vi "Seacrh and Replace String.vi"() -> ()   [LabVIEW 2020]
panel:
  out "Output String":string
  in  "Input String":string="My Self [Fisrt Name] [Last Name]  , My Age is [Age] , My Native Place is [Place]"
  in  "Stop Button":bool
  # "OverView :"
  # "Note :"
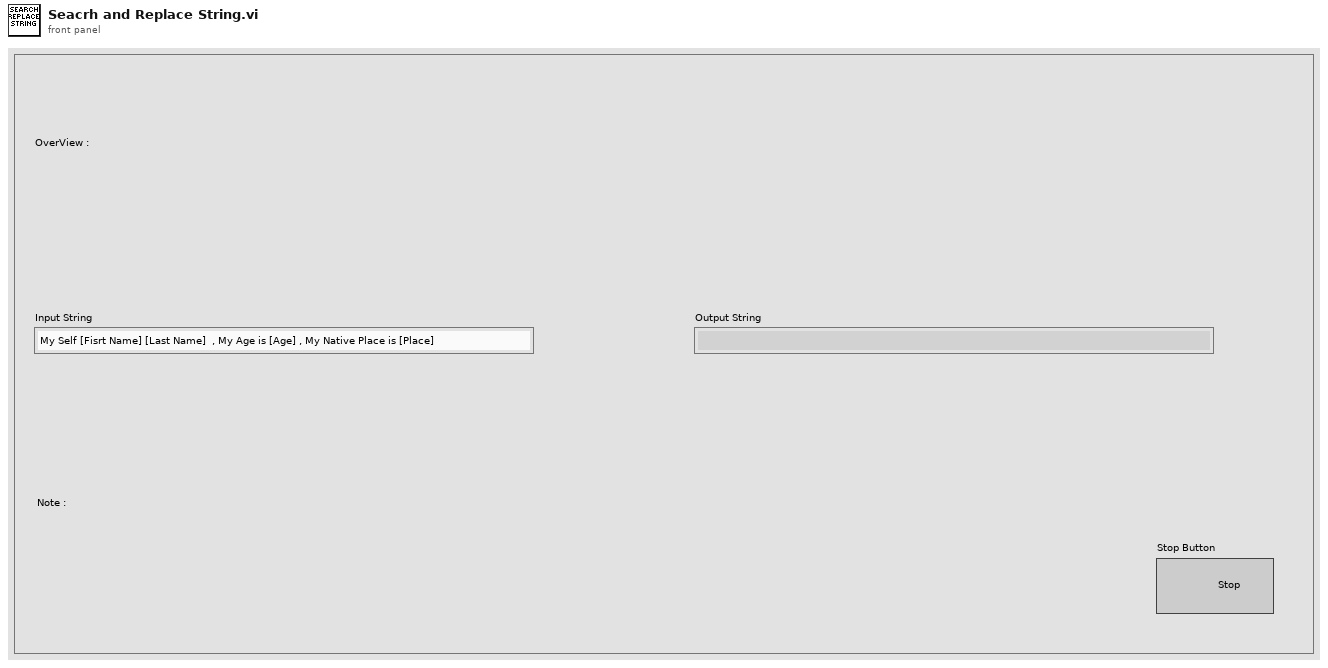
[diagram p1: front panel]
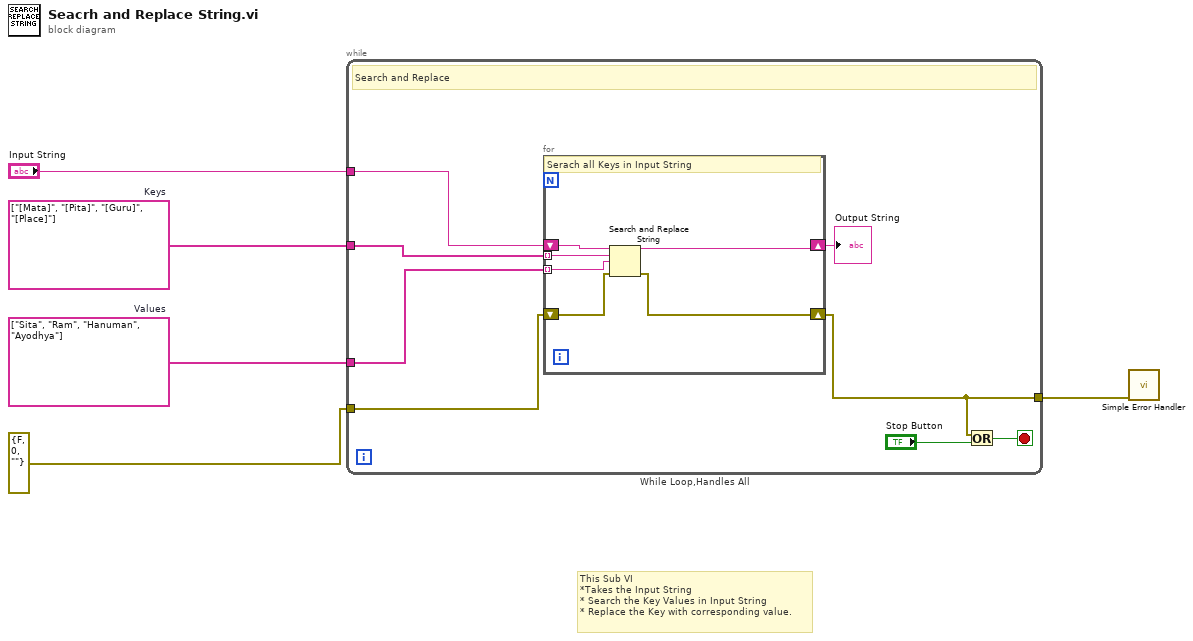
[diagram p0: block diagram]
diagram:
  w3 = string[] ["Sita", "Ram", "Hanuman", "Ayodhya"]  # Values
  w5 = string[] ["[Mata]", "[Pita]", "[Guru]", "[Place]"]  # Keys
  # "This Sub VI\n*Takes the Input String \n* Search the Key Values in Input String \n* Replace the Key with corresponding value."
  n1 = while "While Loop,Handles All" {
    tunnel: w5 -> [w10]
    tunnel: "Input String" -> [w11]
    tunnel: w3 -> [w9]
    tunnel: errorcluster {"status"=FALSE, "code"=0, "source"=""} ("error constant") -> [w8]
    tunnel: [w6] -> w1
    stop <- w12 stop-if-true
    # "Search and Replace"
    n2 = for {
      tunnel: w10 -> [w18] mode=indexing
      tunnel: w9 -> [w17] mode=indexing
      shift-right: [w15] -> w6
      shift-left: w8 -> [w16]
      shift-right: [w14] -> w7
      shift-left: w11 -> [w19]
      # "Serach all Keys in Input String"
      n3 = Search and Replace String(input string=w19, search string=w18, replace string=w17, error in=w16) -> (result string=w14:string, error out=w15:errorcluster)  [unwired: 4 in, 2 out]
    }
    "Output String" <- w7
    n4 = Or(x=w6, y="Stop Button") -> (x .or. y?=w12:bool)
  }
  n5 = call <vilib>:"Simple Error Handler.vi"("error in (no error)"=w1) -> ()  [unwired: 4 in, 5 out]
